vi "Check Expiry.vi"(6 "Now":timestamp, 8 "error in (no error)":errorcluster, 10 "Target Path":string, 11 "Caching in":refnum<class "Caching.lvclass">) -> (0 "error out":errorcluster, 1 "From Cache?":bool, 2 "Response":refnum<class "Response.lvclass">, 3 "Caching out":refnum<class "Caching.lvclass">)   [LabVIEW 2020, in "HTTP Server.lvlib" / "Caching.lvclass"]
uses:
  Caching.lvclass
  Caching.lvclass/Caching.ctl
  lv-http-util/HTTP Utils/Response/Response.lvclass
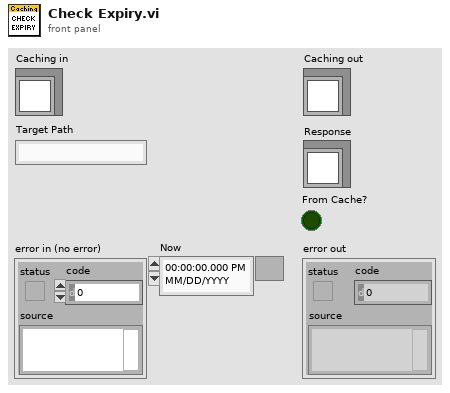
[diagram p1: front panel]
types:
  T1 = typedef "HTTP Server.lvlib/Caching.lvclass/Cache Item.ctl" = cluster{"ID":string, "File":bool, "Path":path, "Value":string, "Created":timestamp, "Expires":timestamp}
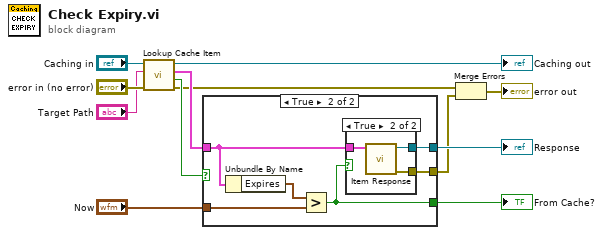
[diagram p0: block diagram]
diagram:
  n1 = call "Lookup Cache Item.vi"("error in (no error)"="error in (no error)", "ID"="Target Path", "Caching in"="Caching in") -> ("error out"=w4:errorcluster, "Found?"=w9:bool, "Cache Item"=w8:T1, "Caching out"=→"Caching out":refnum<class "Caching.lvclass">)  [unwired: 5 in]
  n2 = case shown="True" w9 {
    tunnel: w8 -> [_ w16]
    tunnel: "Now" -> [_ w18]
    tunnel: [_ w15] -> w6
    tunnel: [_ w14] -> w5
    tunnel: [_ w13] -> w3
    frame False {
    }
    frame True {
      n3 = Unbundle By Name(w16) -> ("Expires"=w17:timestamp)
      n4 = Greater?(x=w17, y=w18) -> (0:w15:bool)
      n5 = case shown="True" w15 {
        tunnel: w16 -> [_ w21]
        tunnel: [_ w20] -> w14
        tunnel: [_ w19] -> w13
        frame False {
        }
        frame True {
          n6 = call "Item Response.vi"("Cache Item"=w21) -> ("error out"=w19:errorcluster, "Response"=w20:refnum<class "Response.lvclass">)  [unwired: 9 in]
        }
      }
    }
  }
  "Response" <- w5
  "From Cache?" <- w6
  n7 = Merge Errors(w4, w3) -> (→"error out":errorcluster)
